vi "ROI entry-ROI MotorZ adjustment dialogue.vi"() -> (3 "Cancelled (Left button pressed)":bool)   [LabVIEW 2013]
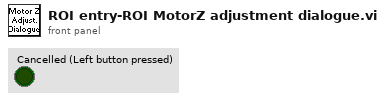
[diagram p1: front panel]
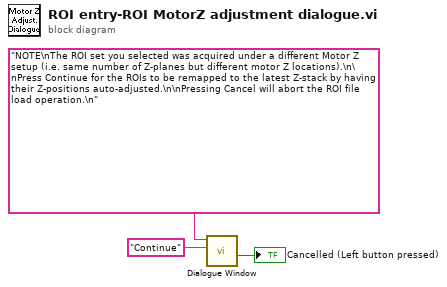
[diagram p0: block diagram]
diagram:
  n1 = call "Dialogue Window.vi"("Caption-Right button (OK)"="Continue", "Message string"="NOTE\nThe ROI set you selected was acquired under a different Motor Z setup (i.e. same number of Z-planes but different motor Z locations).\n\nPress Continue for the ROIs to be remapped to the latest Z-stack by having their Z-positions auto-adjusted.\n\nPressing Cancel will abort the ROI file load operation.\n") -> ("Cancelled (Left button pressed)"=→"Cancelled (Left button pressed)":bool)  [unwired: 7 in, 2 out]
